vi "sub_Set Error Log Path.vi"(8 "error in (no error)":errorcluster, 11 "Path":path) -> (0 "error out":errorcluster)   [LabVIEW 2016, in "System.lvlib"]
uses:
  System.lvlib
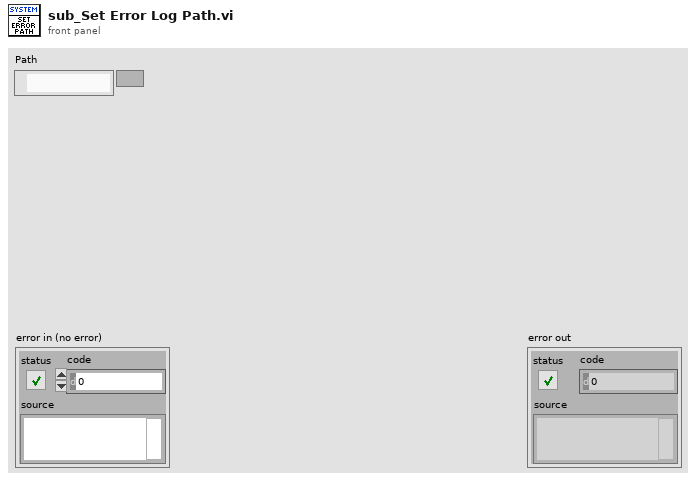
[diagram p1: front panel]
types:
  T1 = typedef "System.lvlib/Control_Variant Data Reference.ctl" = refnum<data-value>
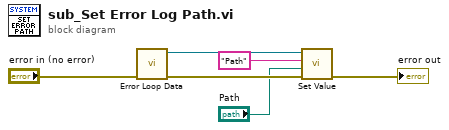
[diagram p0: block diagram]
diagram:
  n1 = call "Error Loop Data.vi"("error in (no error)"="error in (no error)") -> ("error out"=w5:errorcluster, "Error Data Reference"=w6:T1)  [unwired: 9 in]
  n2 = call "Set Value.vi"("error in (no error)"=w5, "Value"="Path", "Name"="Path", "Data Reference"=w6) -> ("error out"=→"error out":errorcluster)  [unwired: 7 in]
